vi "create_from_existing.vi"(10 "Dataset":refnum<class "dataset.lvclass">) -> (3 "Existing Target":refnum<class "target.lvclass">)   [LabVIEW 2020, in "datasources.lvlib" / "target.lvclass"]
uses:
  dataset/dataset.lvclass
  target.lvclass
  target.lvclass/target.ctl
  properties.set.vi
  labels.set.vi
  dataset.set.vi
  channelConfig.set.vi
  workspace.set.vi
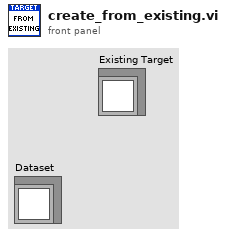
[diagram p1: front panel]
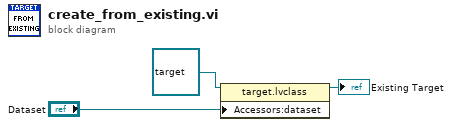
[diagram p0: block diagram]
diagram:
  n1 = property class="target.lvclass"(reference=refnum<class "target.lvclass"> refnum ("Target"), "Accessors:dataset"="Dataset") -> (reference out=→"Existing Target":refnum<class "target.lvclass">)  [unwired: 1 in, 1 out]
